vi "Case Example 022113.vi"() -> ()   [LabVIEW 2012]
panel:
  in  "Numeric 2":i32
  out "Numeric":dbl
  in  "Knob":dbl(knob) scale=0.0..10.0
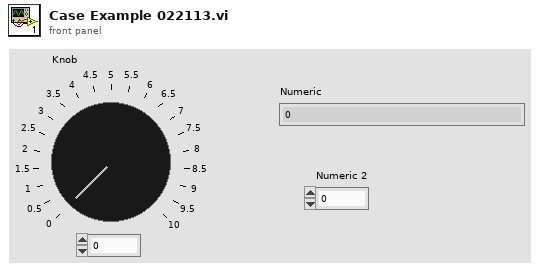
[diagram p1: front panel]
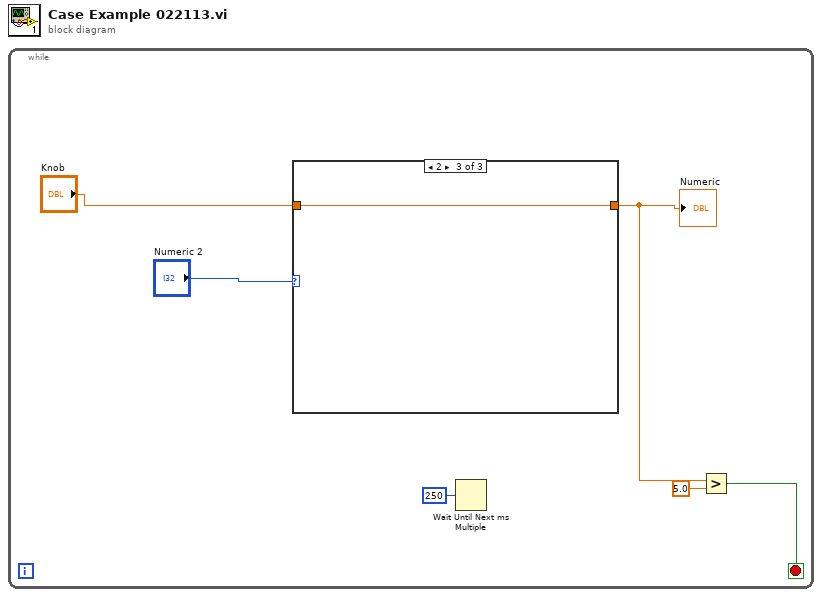
[diagram p0: block diagram]
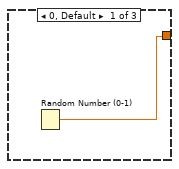
[diagram p2: hidden frame]
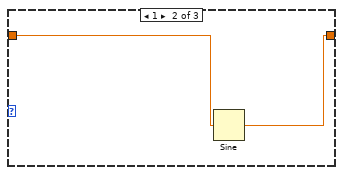
[diagram p3: hidden frame]
diagram:
  n1 = while {
    stop <- w2 stop-if-true
    n2 = case shown="2" "Numeric 2" {
      tunnel: "Knob" -> [_ w9 w10]
      tunnel: [w7 w8 w10] -> w4
      frame 0, Default {
        n3 = Random Number (0-1)() -> (number: 0 to 1=w7:dbl)
      }
      frame 1 {
        n4 = Sine(x=w9) -> (sin(x)=w8:dbl)
      }
      frame 2 {
      }
    }
    "Numeric" <- w4
    n5 = Wait Until Next ms Multiple(millisecond multiple=u32 250) -> ()  [unwired: 1 out]
    n6 = Greater?(x=w4, y=5.0) -> (0:w2:bool)
  }
